vi "Send Channel Settings.vi"(8 "error in":errorcluster, 11 "5105 in":refnum<class "5105.lvclass">) -> (0 "error out":errorcluster, 3 "5105 out":refnum<class "5105.lvclass">)   [LabVIEW 2019, in "5105.lvlib" / "5105.lvclass"]
uses:
  5105.lvclass
  C:/Users/Public/Documents/Development/builds/Instruments/Oscilloscope.lvlibp/Oscilloscope.lvclass
  5105.lvclass/5105.ctl
  builds/Instruments/Oscilloscope.lvlibp/Accessors/Read Channel Settings.vi
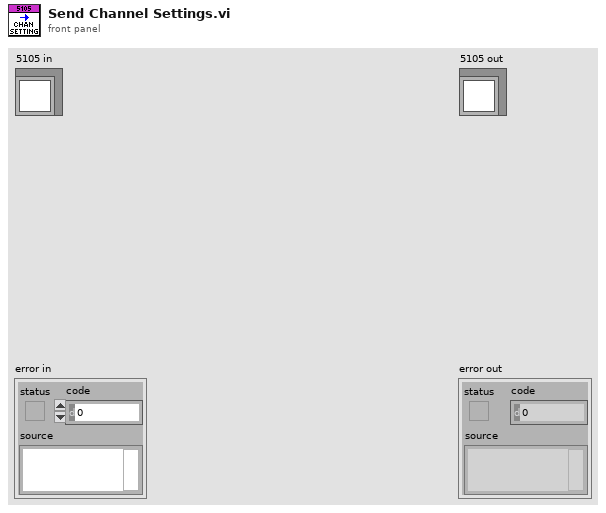
[diagram p1: front panel]
types:
  T1 = typedef "Oscilloscope.lvlibp/Oscilloscope.lvclass/Channel Settings.ctl" = cluster{"Amplitude":dbl, "Vertical Coupling":T2, "Probe Attenuation":dbl, "Enable?":bool, "Maximum Input Frequency":dbl, "Input Impedance":u16, "Timeout (s)":dbl}
  T2 = typedef "Oscilloscope.lvlibp/Oscilloscope.lvclass/Vertical Coupling.ctl" = enum16{"AC", "DC", "Ground"}
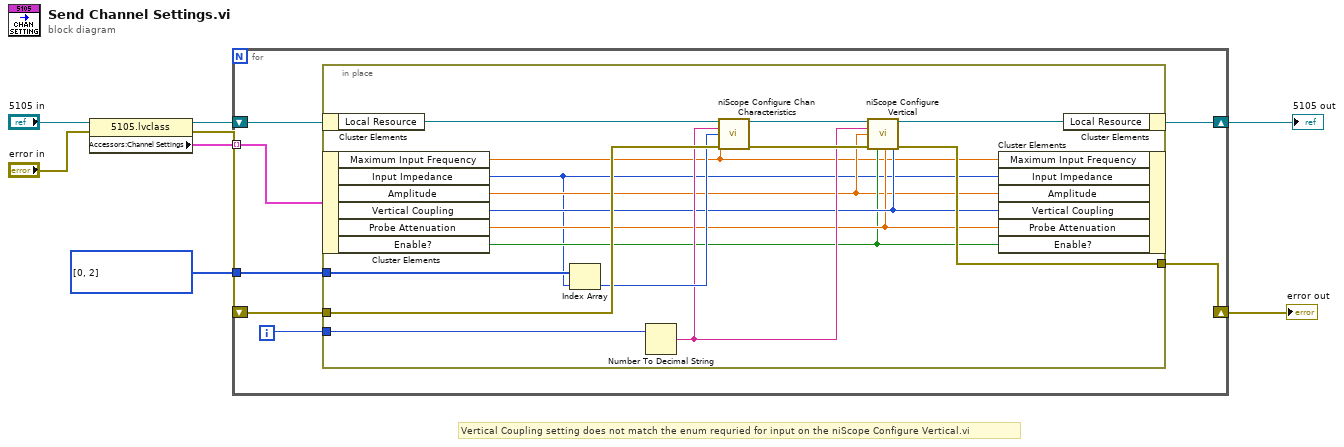
[diagram p0: block diagram]
diagram:
  w1 = u32[] [0, 2] items=["1 mega ohm"=0, "50 ohms"=2]
  # "Vertical Coupling setting does not match the enum requried for input on the niScope Configure Vertical.vi"
  n1 = property class="5105.lvclass"(reference="5105 in", error in="error in") -> (reference out=w5:refnum<class "5105.lvclass">, error out=w4:errorcluster, "Accessors:Channel Settings"=w6:T1[])
  n2 = for {
    tunnel: w6 -> [w9] mode=indexing
    shift-right: [w12] -> w2
    shift-left: w5 -> [w15]
    shift-right: [w13] -> w3
    shift-left: w4 -> [w14]
    tunnel: w1 -> [w10]
    i -> [w11]
    n3 = in-place {
      in-place-border: w14 -> [w26]
      in-place-border: [w30] -> w13
      in-place-border: w11 -> [w25]
      in-place-border: w10 -> [w24]
      n4 = in-place-cluster #1(w15) -> ("Local Resource"=w27:refnum<k15>)
      n5 = in-place-cluster #2(w9) -> ("Maximum Input Frequency"=w16:dbl, "Input Impedance"=w17:u16, "Amplitude"=w18:dbl, "Vertical Coupling"=w21:T2, "Probe Attenuation"=w20:dbl, "Enable?"=w19:bool)
      n6 = Index Array(array=w24, index=w17) -> (element=w23:u32)
      n7 = Number To Decimal String(number=w25) -> (decimal integer string=w22:string)  [unwired: 1 in]
      n8 = call <instrlib>:"niScope Configure Chan Characteristics.vi"("instrument handle"=w27, "channels"=w22, "input impedance"=w23, "maximum input frequency"=w16, "error in"=w26) -> ("instrument handle out"=w29:refnum<k15>, "error out"=w28:errorcluster)  [unwired: 9 in]
      n9 = call <instrlib>:"niScope Configure Vertical.vi"("instrument handle"=w29, "probe attenuation"=w20, "vertical coupling"=w21, "channels"=w22, "vertical range"=w18, "error in"=w28, "channel enabled"=w19) -> ("instrument handle out"=w31:refnum<k15>, "error out"=w30:errorcluster)  [unwired: 7 in]
      n10 = in-place-cluster #2("Maximum Input Frequency"=w16, "Input Impedance"=w17, "Amplitude"=w18, "Vertical Coupling"=w21, "Probe Attenuation"=w20, "Enable?"=w19) -> ()  [unwired: 1 out]
      n11 = in-place-cluster #1("Local Resource"=w31) -> (w12:refnum<class "5105.lvclass">)
    }
  }
  "error out" <- w3
  "5105 out" <- w2
